vi "Finish.vi"   [LabVIEW 2017]
doc: "This VI is called during exit. It can be used to close I/O refnums, save collected data, etc."
uses:
  <vilib>/Rock Robotics/WPI/Utilities/WPI_GetSetVariantRefNum.vi
types:
  T1 = typedef "WPI_SwitchDevRef.ctl" = cluster{"DevStatus":errorcluster, "DIO Channel":T2, "CntIndex":T3, "Normally Closed":bool}
  T2 = typedef "FPGA_DIOChannel.ctl" = enum8{"DIO 0", "DIO 1", "DIO 2", "DIO 3", "DIO 4", "DIO 5", "DIO 6", "DIO 7", "DIO 8", "DIO 9", "DIO MXP 0", "DIO MXP 1", "DIO MXP 2", "DIO MXP 3", "DIO MXP 4", "DIO MXP 5", "DIO MXP 6", "DIO MXP 7", "DIO MXP 8", "DIO MXP 9", "DIO MXP 10", "DIO MXP 11", "DIO MXP 12", "DIO MXP 13", "DIO MXP 14", "DIO MXP 15", "SPI Port CS1", "SPI Port CS2", "SPI Port CS3", "SPI Port MISO", "SPI Port MOSI", "Invalid"}
  T3 = typedef "FPGA_CounterCtrSystemIndex.ctl" = enum8{"Ctr 0", "Ctr 1", "Ctr 2", "Ctr 3", "Ctr 4", "Ctr 5", "Ctr 6", "Ctr 7", "Invalid"}
  T4 = typedef "WPI_JoystickDevRef.ctl" = cluster{"Device":T5}
  T5 = typedef "WPI_JoystickDeviceEnum.ctl" = enum16{"USB 0", "USB 1", "USB 2", "USB 3", "USB 4", "USB 5"}
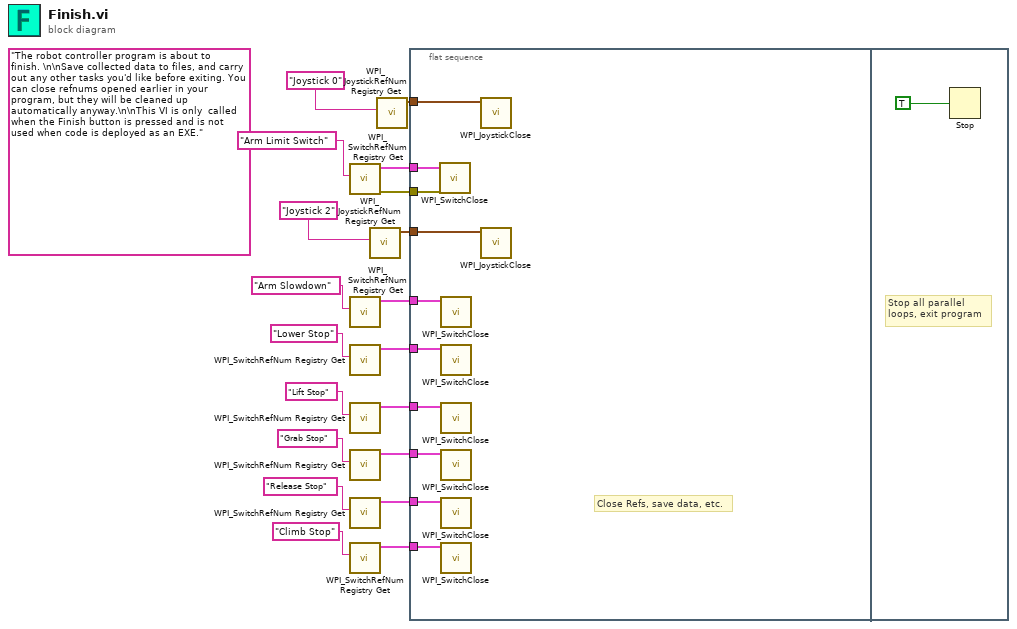
[diagram p0: block diagram]
diagram:
  (unwired) "The robot controller program is about to finish. \n\nSave collected data to files, and carry out any other tasks you'd like before exiting. You can close refnums opened earlier in your program, but they will be cleaned up automatically anyway.\n\nThis VI is only  called when the Finish button is pressed and is not used when code is deployed as an EXE."
  n1 = call <vilib>:"WPI_SwitchRefNum Registry Get.vi"("refnum name"="Arm Limit Switch") -> ("error out"=w2:errorcluster, "SwitchDevRef"=w1:T1)  [unwired: 9 in]
  n2 = call <vilib>:"WPI_SwitchRefNum Registry Get.vi"("refnum name"="Arm Slowdown") -> ("SwitchDevRef"=w14:T1)  [unwired: 9 in, 1 out]
  n3 = call <vilib>:"WPI_SwitchRefNum Registry Get.vi"("refnum name"="Lower Stop") -> ("SwitchDevRef"=w13:T1)  [unwired: 9 in, 1 out]
  n4 = call <vilib>:"WPI_SwitchRefNum Registry Get.vi"("refnum name"="Lift Stop") -> ("SwitchDevRef"=w10:T1)  [unwired: 9 in, 1 out]
  n5 = call <vilib>:"WPI_SwitchRefNum Registry Get.vi"("refnum name"="Grab Stop") -> ("SwitchDevRef"=w5:T1)  [unwired: 9 in, 1 out]
  n6 = call <vilib>:"WPI_SwitchRefNum Registry Get.vi"("refnum name"="Release Stop") -> ("SwitchDevRef"=w6:T1)  [unwired: 9 in, 1 out]
  n7 = call <vilib>:"WPI_SwitchRefNum Registry Get.vi"("refnum name"="Climb Stop") -> ("SwitchDevRef"=w9:T1)  [unwired: 9 in, 1 out]
  n8 = call <vilib>:"WPI_JoystickRefNum Registry Get.vi"("refnum name"="Joystick 2") -> ("JoystickDevRef"=w16:T4)  [unwired: 1 in, 9 out]
  n9 = call <vilib>:"WPI_JoystickRefNum Registry Get.vi"("refnum name"="Joystick 0") -> ("JoystickDevRef"=w18:T4)  [unwired: 1 in, 9 out]
  n10 = flat-sequence {
    tunnel: w18 -> [w29]
    tunnel: w16 -> [w28]
    tunnel: w14 -> [w27]
    tunnel: w13 -> [w26]
    tunnel: w10 -> [w25]
    tunnel: w5 -> [w22]
    tunnel: w6 -> [w23]
    tunnel: w9 -> [w24]
    tunnel: w2 -> [w21]
    tunnel: w1 -> [w20]
    frame #0 {
      # "Close Refs, save data, etc."
      n11 = call <vilib>:"WPI_SwitchClose.vi"("error in (no error)"=w21, "SwitchDevRef"=w20) -> ()  [unwired: 9 in, 1 out]
      n12 = call <vilib>:"WPI_SwitchClose.vi"("SwitchDevRef"=w27) -> ()  [unwired: 10 in, 1 out]
      n13 = call <vilib>:"WPI_SwitchClose.vi"("SwitchDevRef"=w26) -> ()  [unwired: 10 in, 1 out]
      n14 = call <vilib>:"WPI_SwitchClose.vi"("SwitchDevRef"=w25) -> ()  [unwired: 10 in, 1 out]
      n15 = call <vilib>:"WPI_SwitchClose.vi"("SwitchDevRef"=w22) -> ()  [unwired: 10 in, 1 out]
      n16 = call <vilib>:"WPI_SwitchClose.vi"("SwitchDevRef"=w23) -> ()  [unwired: 10 in, 1 out]
      n17 = call <vilib>:"WPI_SwitchClose.vi"("SwitchDevRef"=w24) -> ()  [unwired: 10 in, 1 out]
      n18 = call <vilib>:"WPI_JoystickClose.vi"("JoystickDevRef"=w29) -> ()  [unwired: 11 out]
      n19 = call <vilib>:"WPI_JoystickClose.vi"("JoystickDevRef"=w28) -> ()  [unwired: 11 out]
    }
    frame #1 {
      # "Stop all parallel\nloops, exit program"
      n20 = Stop(stop? (T)=TRUE ("Quit")) -> ()
    }
  }
